vi "RelaysName_String.vi"(11 "relay names":string) -> (3 "Array":string[](array[string]))   [LabVIEW 2015]
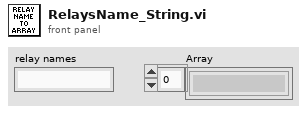
[diagram p1: front panel]
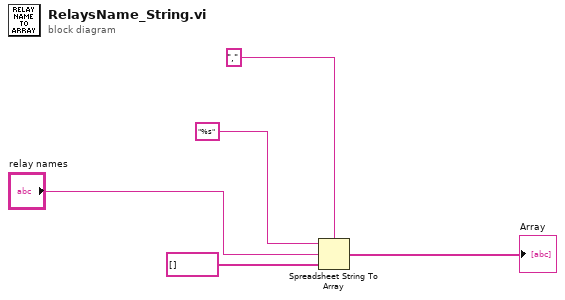
[diagram p0: block diagram]
diagram:
  n1 = Spreadsheet String To Array(delimiter (Tab)=",", format string="%s", spreadsheet string="relay names", array type (2D Dbl)=string[] []) -> (array=→"Array":string[])
